vi "AB_CombinePaths.vi"(10 "target path":path, 11 "localDestPath":path) -> (3 "combined path":path)   [LabVIEW 2020]
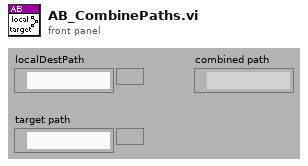
[diagram p1: front panel]
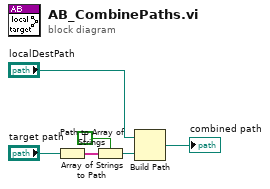
[diagram p0: block diagram]
diagram:
  n1 = Path to Array of Strings(0:"target path") -> (2:w5:string[])  [unwired: 1 out]
  n2 = Array of Strings to Path(0:w5, 1:TRUE ("relative")) -> (2:w2:path)
  n3 = Build Path(base path="localDestPath", name or relative path=w2) -> (appended path=→"combined path":path)
